vi "Display_Controls_Ctrl_Index.vi"(5 "OldVal":variant, 11 "NewVal":variant) -> (4 "Control Ref OUT":refnum<vi>, 8 "Display Controls Out":T1)   [LabVIEW 2014]
uses:
  Type Defs/Display Controls.ctl
panel:
  in  "Display Controls Data Type":T1
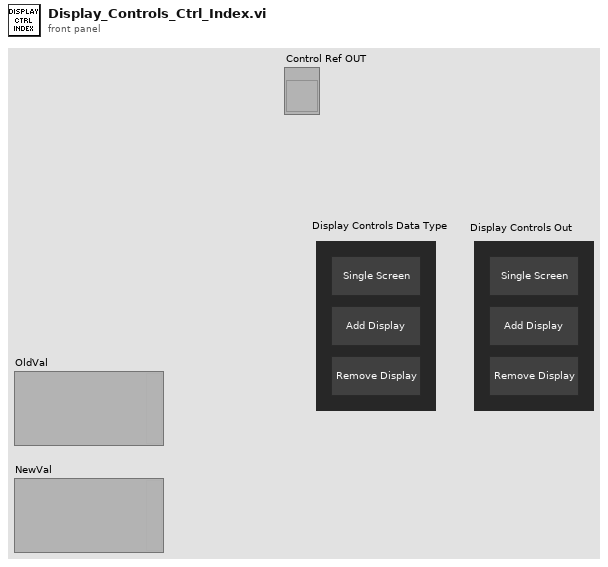
[diagram p1: front panel]
types:
  T1 = typedef "Display Controls.ctl" = cluster{"Remove Display":bool, "Add Display":bool, "Single Screen":bool}
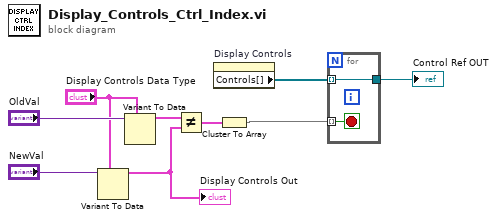
[diagram p0: block diagram]
diagram:
  n1 = Variant To Data(type="Display Controls Data Type", Variant="NewVal") -> (data=w3:T1)  [unwired: 1 in, 1 out]
  "Display Controls Out" <- w3
  n2 = Variant To Data(type="Display Controls Data Type", Variant="OldVal") -> (data=w5:T1)  [unwired: 1 in, 1 out]
  n3 = Not Equal?(x=w5, y=w3) -> (x != y?=w9:T1)
  n4 = property on="Display Controls" class="Clust (strict)"() -> ("Controls[]"=w1:refnum<vi>[])  [unwired: 2 in, 2 out]
  n5 = Cluster To Array(cluster=w9) -> (array=w6:bool[])
  n6 = for {
    tunnel: w6 -> [w10] mode=indexing
    tunnel: w1 -> [w11] mode=indexing
    tunnel: [w11] -> w4
    stop <- w10 stop-if-true
  }
  "Control Ref OUT" <- w4
